vi "Configure Power Present.vi"(7 "error in (no error)":errorcluster {"code" format="%.0x"}, 9 "Enabled":i32[](array[numeric])=[0, 0, 0], 10 "instrument handle":refnum<k15>) -> (0 "error out":errorcluster {"code" format="%.0x"}, 1 "EnabledActualSize":i32, 3 "instrument handle out":refnum<k15>)   [LabVIEW 2009, in "Keysight XSAn.lvlib"]
doc: "Configures the carriers for this measurement. It allows spaces to be inserted between carriers. Carriers with the power present parameter set to Yes are carriers, and those with the power present parameter set to No are spaces. Each carrier power present is set to Yes or No.\n\nSupported Models: M9290A, N8973B, N8974B, N8975B, N8976B, N9000A, N9000B, N9010A, N9010B, N9020A, N9020B, N9030A, N9030B, N9038A, N9040B, N9041B, SPN9003A, SPN9026A"
uses:
  <instrlib>/Keysight XSAn/Keysight XSAn.lvlib
  AgXSAn.dll
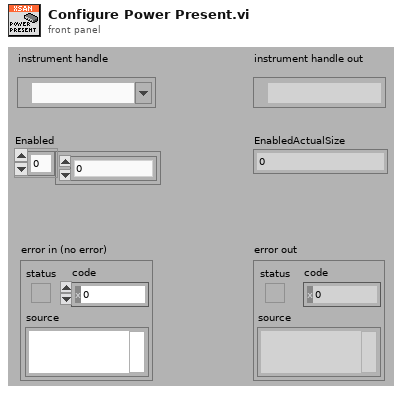
[diagram p1: front panel]
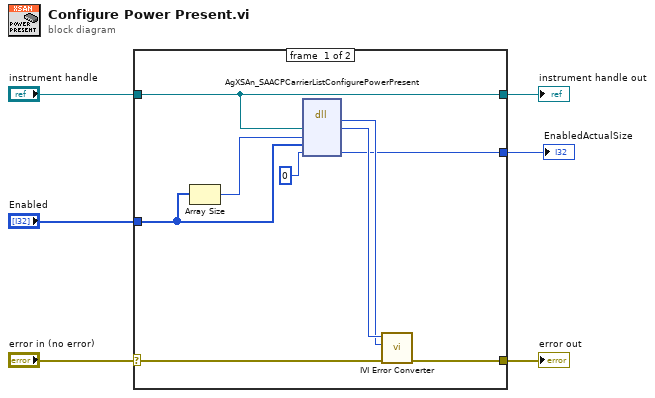
[diagram p0: block diagram]
diagram:
  n1 = case shown="No Error" "error in (no error)" {
    selector: "error in (no error)" -> [w13 w17]
    tunnel: [w12 w17] -> w6
    tunnel: "instrument handle" -> [w9 w16]
    tunnel: [w10 _] -> w3
    tunnel: [w9 w16] -> w2
    tunnel: "Enabled" -> [w8 _]
    frame #0 {
      n2 = Array Size(array=w8) -> (size(s)=w7:i32)
      n3 = dll-call lib="AgXSAn**.dll" fn="AgXSAn_SAACPCarrierListConfigurePowerPresent"("Vi"=w9, "EnabledBufferSize"=w7, "Enabled"=w8, "EnabledActualSize"=0) -> (w14:i32, "Vi"=w15:u32, "EnabledActualSize"=w10:i32)  [unwired: 5 in, 2 out]
      n4 = call <instrlib>:"IVI Error Converter.vi"("error in (no error)"=w13, "IVI error code (0)"=w14, "instrument handle"=w15) -> ("error out"=w12:errorcluster)  [unwired: 7 in, 1 out]
    }
    frame #1 {
    }
  }
  "error out" <- w6
  "instrument handle out" <- w2
  "EnabledActualSize" <- w3
